vi "Parse Tree Parameters.vi"(0 "Custom Device Ref":T1 format="%.0x", 5 "Item Ref in":T1 format="%.0x", 9 "Specified Channel Ref List":T1[](array[typedef]) format="%.0x", 11 "error in":errorcluster, 12 "Timestamp Ref":T1=18446744073709551615 format="%.0x", 13 "Timestamp?":bool) -> (4 "Item Ref out":T1 format="%.0x", 14 "Parameter Driver Data":T2 {"Num Bits" min=1 max=32; "Start Bit" min=8 max=31}, 15 "error out":errorcluster)   [LabVIEW 2017, in "Ballard Arinc-429 System Explorer.lvlib"]
uses:
  System Explorer/Ballard Arinc-429 System Explorer.lvlib
  <vilib>/NI Veristand/Custom Device API/Custom Device Item Ref.ctl
  RT Controls/RT Param Setting.ctl
  Shared/Controls and Global/Start Bit.ctl
  Shared/Controls and Global/Number of Bits.ctl
  <vilib>/NI Veristand/Custom Device API/Get Item Property (I32).vi
  <vilib>/NI Veristand/Custom Device API/Get Item Property (Double).vi
  <vilib>/NI Veristand/Custom Device API/Get Item Property (Boolean).vi
  <vilib>/NI Veristand/Custom Device Tools/Custom Device Utility Library/NI VeriStand - Search for All Items by GUID.vi
  Shared/Controls and Global/Global.vi
  <vilib>/NI Veristand/Custom Device API/Custom Device API.lvlib
  <vilib>/NI Veristand/Custom Device Tools/Custom Device Utility Library/Custom Device Utility Library.lvlib
  Shared/Ballard Arinc-429 Shared.lvlib
  Ballard Arinc-429 Engine.lvlib
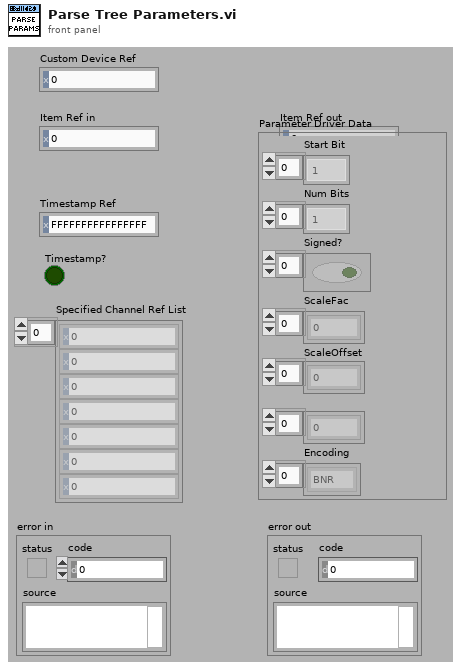
[diagram p1: front panel]
types:
  T1 = typedef "Custom Device API.lvlib/Custom Device Item Ref.ctl" = u64
  T2 = typedef "Ballard Arinc-429 Engine.lvlib/RT Param Setting.ctl" = cluster{"Start Bit":T3[], "Num Bits":T4[], "Signed?":bool[], "ScaleFac":dbl[], "ScaleOffset":dbl[], "Channel FIFO Buffer Index":i32[], "Encoding":enum16{"BNR", "BCD", "Discrete"}[]}
  T3 = typedef "Ballard Arinc-429 Shared.lvlib/Start Bit.ctl" = i32
  T4 = typedef "Ballard Arinc-429 Shared.lvlib/Number of Bits.ctl" = i32
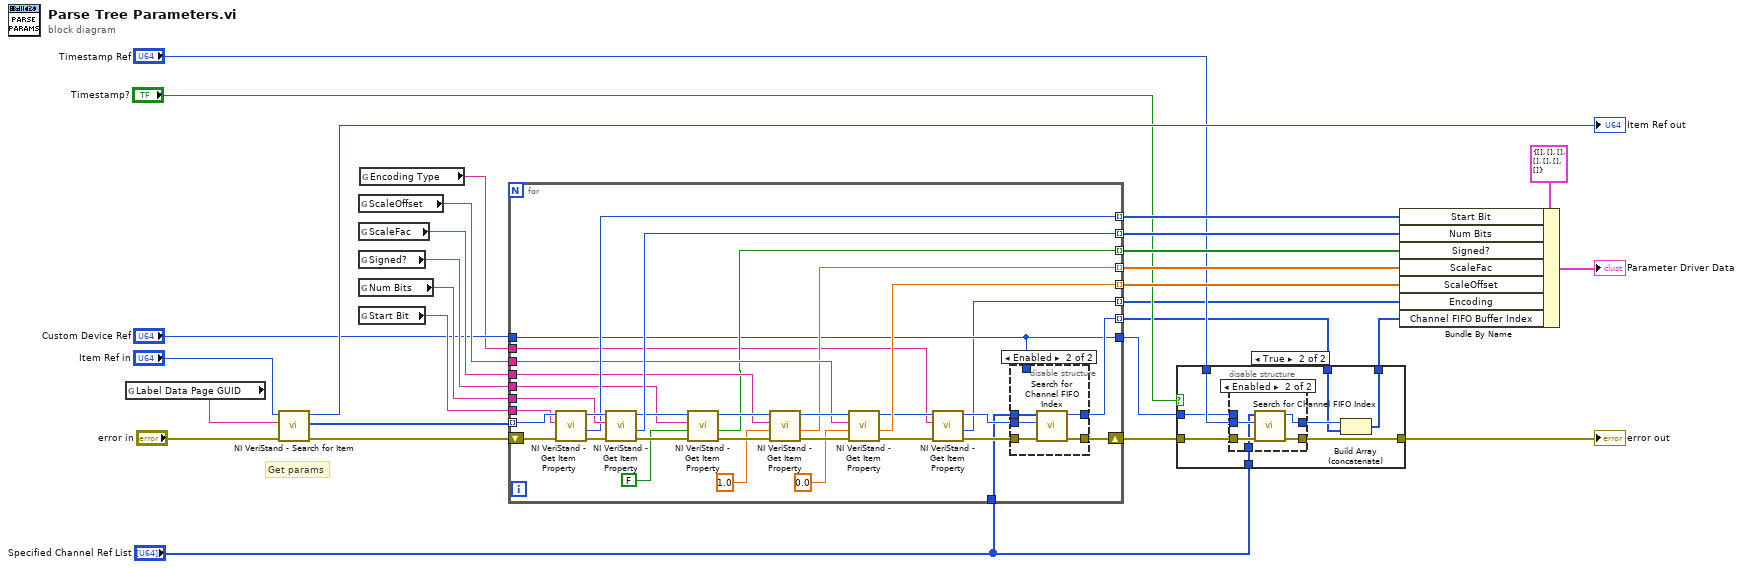
[diagram p0: block diagram]
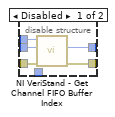
[diagram p3: hidden frame]
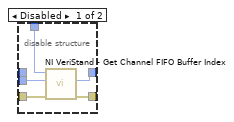
[diagram p4: hidden frame]
diagram:
  # "Get params"
  n1 = global read "Global.vi" "Label Data Page GUID"() -> (w27:string)
  n2 = call-poly <vilib>:"NI VeriStand - Search for Item.vi"("error in"="error in", "Item GUID"=w27, "Section Ref in"="Item Ref in") -> ("error out"=w24:errorcluster, "Item Refs"=w23:T1[], "Section Ref out"=→"Item Ref out":T1)  [unwired: 5 in, 1 out]
  n3 = global read "Global.vi" "ScaleOffset"() -> (w17:string)
  n4 = global read "Global.vi" "ScaleFac"() -> (w18:string)
  n5 = global read "Global.vi" "Signed?"() -> (w19:string)
  n6 = global read "Global.vi" "Num Bits"() -> (w29:string)
  n7 = global read "Global.vi" "Start Bit"() -> (w28:string)
  n8 = global read "Global.vi" "Encoding Type"() -> (w3:string)
  n9 = for {
    shift-right: [w39] -> w10
    shift-left: w24 -> [w62]
    tunnel: w23 -> [w61] mode=indexing
    tunnel: w28 -> [w58]
    tunnel: w29 -> [w57]
    tunnel: [w56] -> w21 mode=indexing
    tunnel: [w55] -> w20 mode=indexing
    tunnel: w19 -> [w48]
    tunnel: w18 -> [w46]
    tunnel: w17 -> [w44]
    tunnel: [w42] -> w16 mode=indexing
    tunnel: [w41] -> w15 mode=indexing
    tunnel: [w40] -> w14 mode=indexing
    tunnel: [w38] -> w5 mode=indexing
    tunnel: "Custom Device Ref" -> [w37]
    tunnel: [w37] -> w6
    tunnel: w3 -> [w32]
    tunnel: [w31] -> w2 mode=indexing
    tunnel: "Specified Channel Ref List" -> [w30]
    n10 = call-poly <vilib>:"NI VeriStand - Get Item Property.vi"("error in (no error)"=w62, "Property Name"=w58, "Item Ref in"=w61) -> ("error out"=w60:errorcluster, "Value"=w56:i32, "Item Ref out"=w59:T1)  [unwired: 5 in, 1 out]
    n11 = call-poly <vilib>:"NI VeriStand - Get Item Property.vi"("error in (no error)"=w60, "Property Name"=w57, "Item Ref in"=w59) -> ("error out"=w49:errorcluster, "Value"=w55:i32, "Item Ref out"=w54:T1)  [unwired: 5 in, 1 out]
    n12 = call-poly <vilib>:"NI VeriStand - Get Item Property.vi"("error in (no error)"=w49, "Default Value"=FALSE, "Property Name"=w48, "Item Ref in"=w54) -> ("error out"=w50:errorcluster, "Value"=w42:bool, "Item Ref out"=w53:T1)  [unwired: 4 in, 1 out]
    n13 = call-poly <vilib>:"NI VeriStand - Get Item Property.vi"("error in (no error)"=w50, "Default Value"=1.0, "Property Name"=w46, "Item Ref in"=w53) -> ("error out"=w51:errorcluster, "Value"=w41:dbl, "Item Ref out"=w52:T1)  [unwired: 4 in, 1 out]
    n14 = call-poly <vilib>:"NI VeriStand - Get Item Property.vi"("error in (no error)"=w51, "Default Value"=0.0, "Property Name"=w44, "Item Ref in"=w52) -> ("error out"=w36:errorcluster, "Value"=w40:dbl, "Item Ref out"=w34:T1)  [unwired: 4 in, 1 out]
    n15 = call-poly <vilib>:"NI VeriStand - Get Item Property.vi"("error in (no error)"=w36, "Property Name"=w32, "Item Ref in"=w34) -> ("error out"=w35:errorcluster, "Value"=w31:i32, "Item Ref out"=w33:T1)  [unwired: 5 in, 1 out]
    n16 = disable-structure shown="Enabled" {
      disable-tunnel: [w67 w68] -> w39
      disable-tunnel: [w66 w72] -> w38
      disable-tunnel: w37 -> [w65 _]
      disable-tunnel: w35 -> [w64 w71]
      disable-tunnel: w33 -> [w63 w70]
      disable-tunnel: w30 -> [_ w69]
      frame Disabled {
        n17 = call <vilib>:"NI VeriStand - Get Channel FIFO Buffer Index.vi"("error in"=w64, "Channel Ref"=w63, "Device Ref in"=w65) -> ("error out"=w67:errorcluster, "Channel FIFO Buffer Index"=w66:i32)  [unwired: 4 in, 3 out]
      }
      frame Enabled {
        n18 = call "Search for Channel FIFO Index.vi"("error in (no error)"=w71, "Item Ref"=w70, "Specified Channel Ref List"=w69) -> ("error out"=w68:errorcluster, "index of element"=w72:i32)  [unwired: 7 in]
      }
    }
  }
  n19 = case shown="True" "Timestamp?" {
    tunnel: w10 -> [w74 w82]
    tunnel: [w74 w81] -> w9
    tunnel: "Timestamp Ref" -> [_ w80]
    tunnel: w6 -> [_ w79]
    tunnel: w5 -> [w73 w77]
    tunnel: [w73 w76] -> w4
    tunnel: "Specified Channel Ref List" -> [_ w75]
    frame False {
    }
    frame True {
      n20 = disable-structure shown="Enabled" {
        disable-tunnel: w82 -> [w87 w91]
        disable-tunnel: [w86 w90] -> w81
        disable-tunnel: w80 -> [w85 w92]
        disable-tunnel: w79 -> [w84 _]
        disable-tunnel: [w83 w89] -> w78
        disable-tunnel: w75 -> [_ w88]
        frame Disabled {
          n21 = call <vilib>:"NI VeriStand - Get Channel FIFO Buffer Index.vi"("error in"=w87, "Channel Ref"=w85, "Device Ref in"=w84) -> ("error out"=w86:errorcluster, "Channel FIFO Buffer Index"=w83:i32)  [unwired: 4 in, 3 out]
        }
        frame Enabled {
          n22 = call "Search for Channel FIFO Index.vi"("error in (no error)"=w91, "Item Ref"=w92, "Specified Channel Ref List"=w88) -> ("error out"=w90:errorcluster, "index of element"=w89:i32)  [unwired: 7 in]
        }
      }
      n23 = Build Array (concatenate)(w78, w77) -> (w76:i32[])
    }
  }
  "error out" <- w9
  n24 = Bundle By Name(cluster=T2 {"Start Bit"=[], "Num Bits"=[], "Signed?"=[], "ScaleFac"=[], "ScaleOffset"=[], "Channel FIFO Buffer Index"=[], "Encoding"=[]} ("Param Setting"), "Start Bit"=w21, "Num Bits"=w20, "Signed?"=w16, "ScaleFac"=w15, "ScaleOffset"=w14, "Encoding"=w2, "Channel FIFO Buffer Index"=w4) -> (→"Parameter Driver Data":T2)
